vi "EEG_2022_040_LabView_3.2.vi"() -> ()   [LabVIEW 2022 SP3]
panel:
  out "Number of Iterations":u32
  out "Current Number":u32
  in  "Number to Match":u32 max=1000 step=1
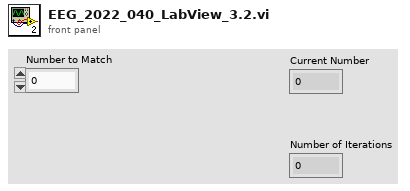
[diagram p1: front panel]
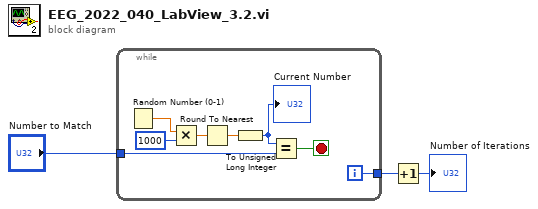
[diagram p0: block diagram]
diagram:
  n1 = while {
    tunnel: "Number to Match" -> [w7]
    tunnel: [w5] -> w1
    i -> [w5]
    stop <- w6 stop-if-true
    n2 = Random Number (0-1)() -> (number: 0 to 1=w11:dbl)
    n3 = Multiply(x=w11, y=1000) -> (x*y=w9:dbl)
    n4 = Round To Nearest(number=w9) -> (nearest integer value=w8:dbl)
    n5 = To Unsigned Long Integer(number=w8) -> (unsigned 32bit integer=w4:u32)
    "Current Number" <- w4
    n6 = Equal?(x=w4, y=w7) -> (x = y?=w6:bool)
  }
  n7 = Increment(x=w1) -> (x+1=→"Number of Iterations":i32)
